vi "SetPanel.vi"(8 "error in (no error)":errorcluster) -> (0 "error out":errorcluster)   [LabVIEW 2019]
uses:
  <vilib>/Utility/miscctls.llb/LVPointTypeDef.ctl
  <vilib>/Utility/miscctls.llb/LVPositionTypeDef.ctl
panel:
  in  "Tab Control":enum32{"Page 1", "Page 2"}(tab)
  in  "$DelayNum_":i32 caption="延遲取像時間(ms)" min=0 step=1
  in  "$DirectionNum_":T1(ring) caption="取料起始位置"
  in  "$ErrtimeNum_":i32 caption="重測次數上限" min=0 step=1
  in  "$ItemDistanceNum_":dbl caption="料件距離(Pixel/mm)" min=0.0 step=0.001 format="%#_4g"
  in  "$Ring":u16(ring) caption="Ring" items=["A", "V", "C"]
  in  "$VType":enum16{"無條件捨去", "四捨五入"}(ring) caption="電壓選取方式"
  in  "$ForceSetBinChk_":bool caption="使用手動參數"
  in  "$Standar VNum_":string caption="標準電壓"
  in  "$VISA resource name":refnum<visa-resource-name>
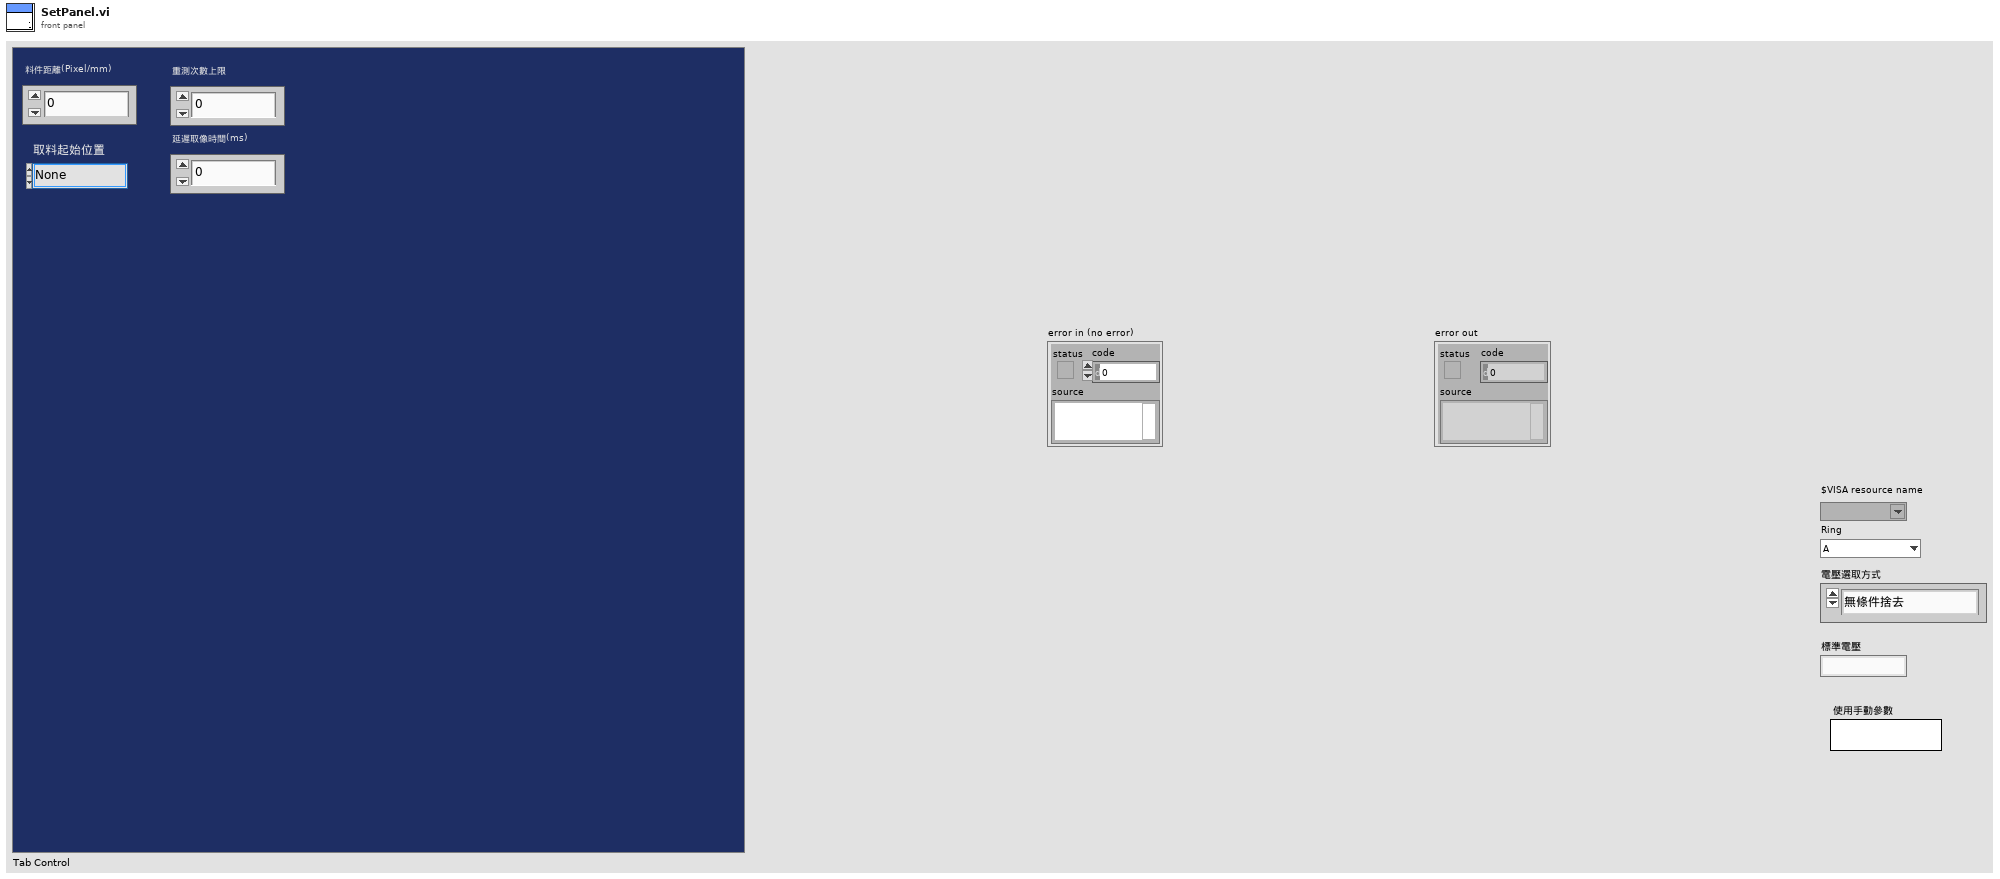
[diagram p1: front panel]
types:
  T1 = enum16{"None", "Image左上", "Image左下", "Image右上", "Image右下"}
  T2 = typedef "LVPositionTypeDef.ctl" = cluster{"Left":i32, "Top":i32}
  T3 = typedef "LVPointTypeDef.ctl" = cluster{"Horizontal":i16, "Vertical":i16}
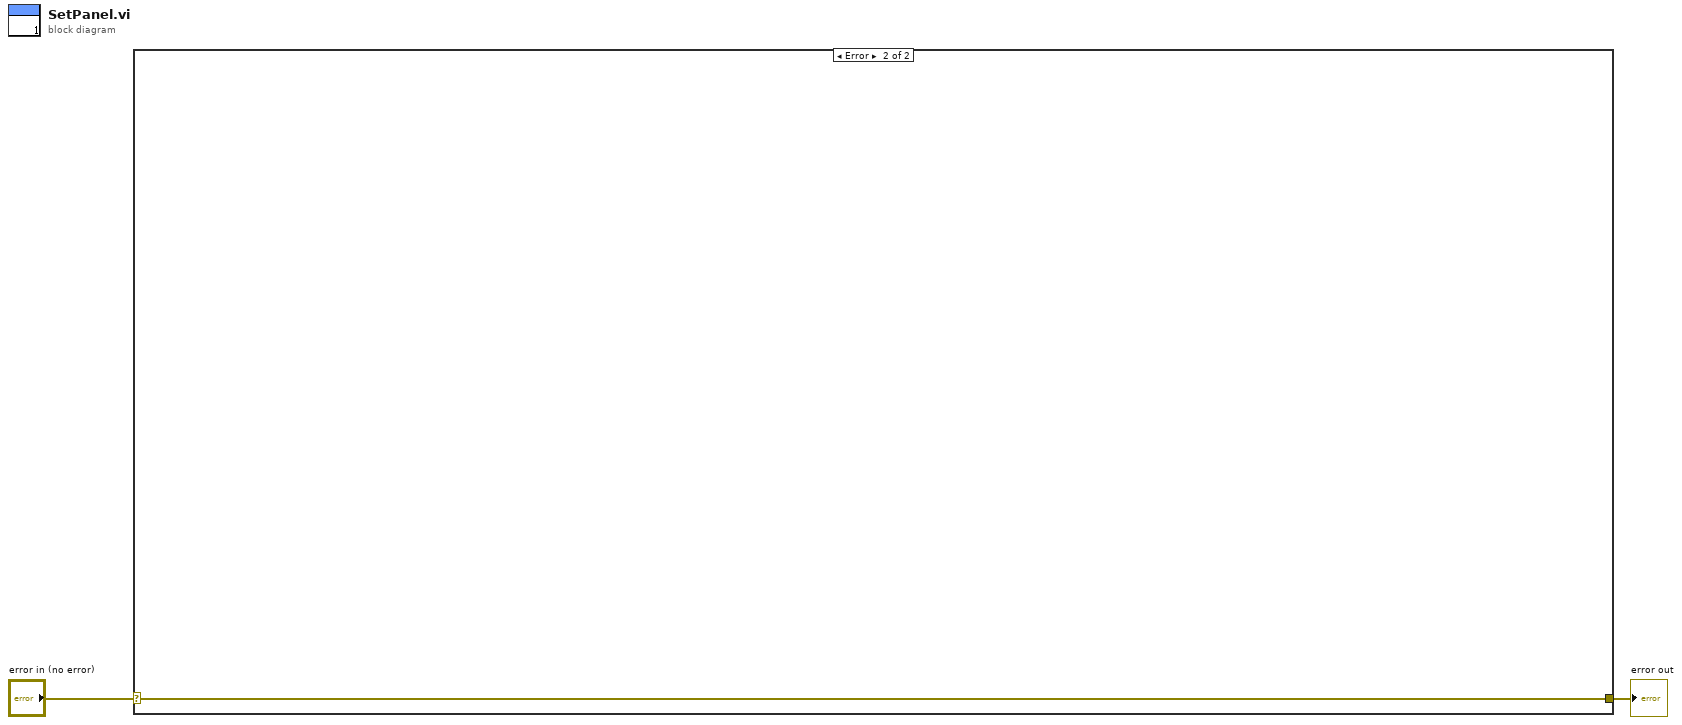
[diagram p0: block diagram]
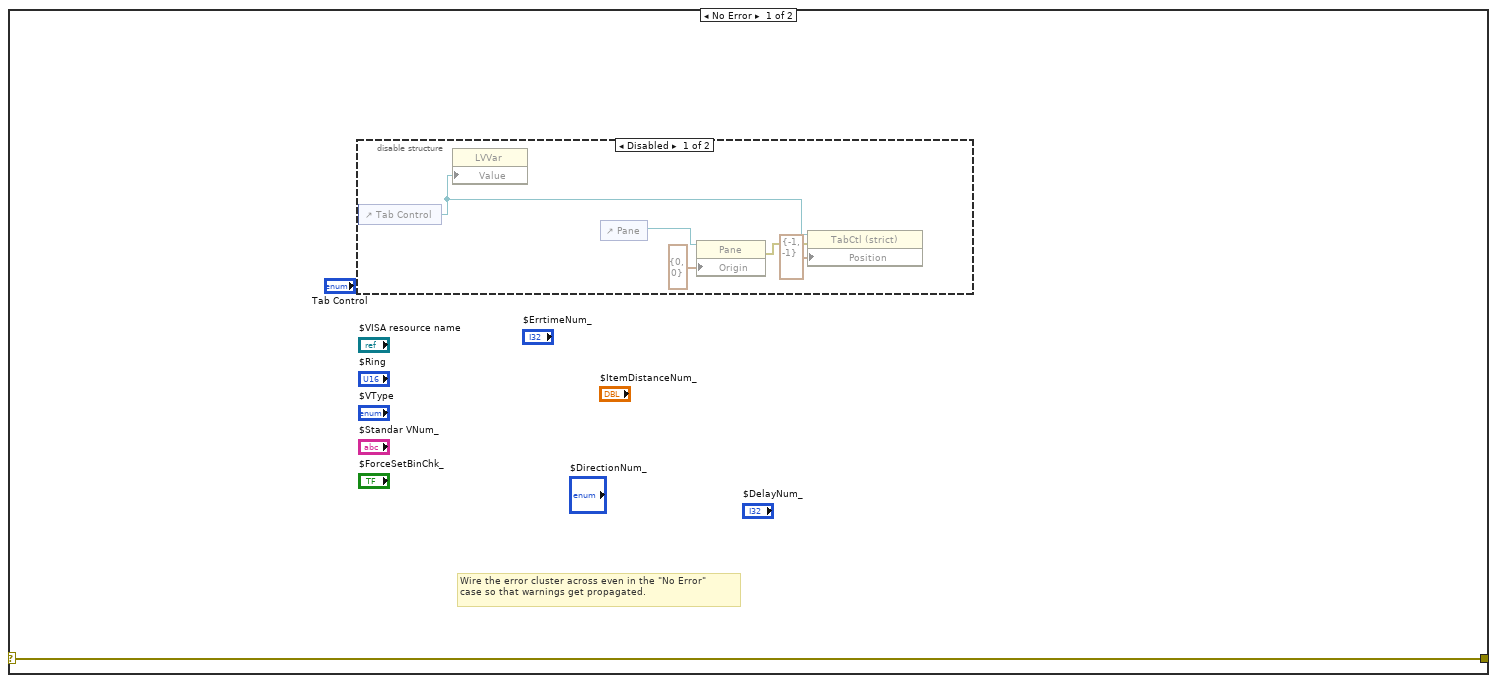
[diagram p2: hidden frame]
diagram:
  n1 = case shown="Error" "error in (no error)" {
    selector: "error in (no error)" -> [w3 w9]
    tunnel: [w3 w9] -> w1
    frame No Error {
      # "Wire the error cluster across even in the \"No Error\"\ncase so that warnings get propagated."
      n2 = disable-structure shown="Disabled" {
        frame Disabled {
          n3 = control-ref of="Tab Control"() -> (w6:refnum<vi>)
          n4 = property class="LVVar"("Value"=w6) -> ()  [unwired: 2 in, 2 out]
          n5 = control-ref of="Pane"() -> (w4:refnum<vi>)
          n6 = property class="Pane"(reference=w4, "Origin"=T3 {"Horizontal"=0, "Vertical"=0}) -> (error out=w7:errorcluster)  [unwired: 1 in, 1 out]
          n7 = property class="TabCtl (strict)"(reference=w6, error in=w7, "Position"=T2 {"Left"=-1, "Top"=-1}) -> ()  [unwired: 2 out]
        }
        frame Enabled {
        }
      }
    }
    frame Error {
    }
  }
  "error out" <- w1
